vi "VerifIdleAsync.vi"(8 "error in (no error)":errorcluster, 11 "S4GUI in":refnum<class "S4GUI.lvclass">) -> (0 "error out":errorcluster, 3 "S4GUI out":refnum<class "S4GUI.lvclass">)   [LabVIEW 2018, in "S4GUI.lvclass"]
uses:
  S4GUI.lvclass
  S4GUI.lvclass/S4GUI.ctl
  Acquisition/Acquisition.lvclass
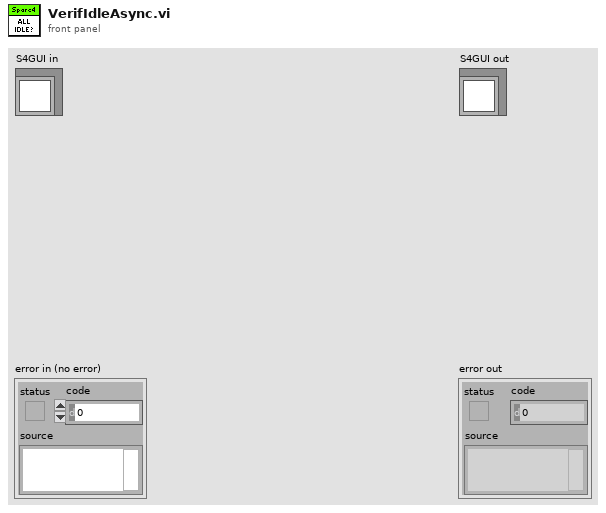
[diagram p1: front panel]
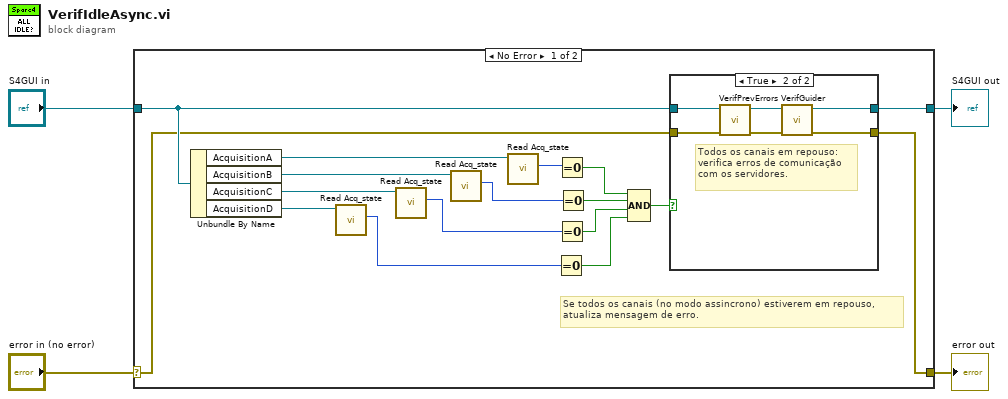
[diagram p0: block diagram]
diagram:
  n1 = case shown="No Error" "error in (no error)" {
    selector: "error in (no error)" -> [w6 w31]
    tunnel: [w5 w31] -> w3
    tunnel: [w7 w30] -> w1
    tunnel: "S4GUI in" -> [w8 w30]
    frame No Error {
      # "Se todos os canais (no modo assincrono) estiverem em repouso,\natualiza mensagem de erro."
      n2 = Unbundle By Name(w8) -> ("AcquisitionA"=w21:refnum<class "Acquisition.lvclass">, "AcquisitionB"=w20:refnum<class "Acquisition.lvclass">, "AcquisitionC"=w19:refnum<class "Acquisition.lvclass">, "AcquisitionD"=w18:refnum<class "Acquisition.lvclass">)
      n3 = call-dynamic "Read Acq_state.vi"("Acquisition in"=w18) -> ("Acq_state"=w14:u32)  [unwired: 8 in, 2 out]
      n4 = call-dynamic "Read Acq_state.vi"("Acquisition in"=w19) -> ("Acq_state"=w15:u32)  [unwired: 8 in, 2 out]
      n5 = call-dynamic "Read Acq_state.vi"("Acquisition in"=w20) -> ("Acq_state"=w16:u32)  [unwired: 8 in, 2 out]
      n6 = call-dynamic "Read Acq_state.vi"("Acquisition in"=w21) -> ("Acq_state"=w17:u32)  [unwired: 8 in, 2 out]
      n7 = Equal To 0?(x=w14) -> (x = 0?=w10:bool)
      n8 = Equal To 0?(x=w17) -> (x = 0?=w13:bool)
      n9 = Equal To 0?(x=w15) -> (x = 0?=w11:bool)
      n10 = Equal To 0?(x=w16) -> (x = 0?=w12:bool)
      n11 = Compound Arithmetic op=AND(w13, w12, w11, w10) -> (w9:bool)
      n12 = case shown="True" w9 {
        tunnel: w8 -> [w23 w29]
        tunnel: [w23 w27] -> w7
        tunnel: w6 -> [w22 w26]
        tunnel: [w22 w24] -> w5
        frame False {
          # "Algum canal adquirindo...\nnão deve interferir em \n\"Error Msg\"."
        }
        frame True {
          # "Todos os canais em repouso:\nverifica erros de comunicação\ncom os servidores."
          n13 = call-dynamic "VerifPrevErrors.vi"("error in (no error)"=w26, "S4GUI in"=w29) -> ("error out"=w25:errorcluster, "S4GUI out"=w28:refnum<class "S4GUI.lvclass">)  [unwired: 8 in]
          n14 = call-dynamic "VerifGuider.vi"("error in (no error)"=w25, "S4GUI in"=w28) -> ("error out"=w24:errorcluster, "S4GUI out"=w27:refnum<class "S4GUI.lvclass">)  [unwired: 8 in]
        }
      }
    }
    frame Error {
    }
  }
  "error out" <- w3
  "S4GUI out" <- w1
